vi "MecaOdometry_Update.vi"(8 "WheelSpeeds":T8 {"RearRightSpeed" format="%19.3f"; "RearLeftSpeed" format="%19.3f"; "FrontRightSpeed" format="%19.3f"; "FrontLeftSpeed" format="%19.3f"}, 9 "GyroAngle":T4={"VALUE"=0.0, "COS"=1.0, "SIN"=0.0} {"SIN" format="%13.4f"; "COS" format="%13.4f"; "VALUE" format="%13.4f"}, 10 "Time":dbl=-1.0 format="%33.4f", 11 "in MECA_DRIVE_ODOMETRY":T1={"POSE"={"TRANSLATION"={"X"=0.0, "Y"=0.0}, "ROTATION"={"VALUE"=0.0, "COS"=1.0, "SIN"=0.0}}, "PrevTime"=0.0, "GyroOffset"={"VALUE"=0.0, "COS"=0.0, "SIN"=0.0}, "PreviousAngle"={"VALUE"=0.0, "COS"=0.0, "SIN"=0.0}, "Kinematics"={"FrontLeft"={"X"=0.0, "Y"=0.0}, "FrontRight"={"X"=0.0, "Y"=0.0}, "RearLeft"={"X"=0.0, "Y"=0.0}, "RearRight"={"X"=0.0, "Y"=0.0}, "InverseKinematics"=[[0.0, 1.0, -1.0, 0.0], [0.0, 1.0, 1.0, 0.0], [0.0, 1.0, 1.0, 0.0], [0.0, 1.0, -1.0, 0.0]], "ForwardKinematics"=[[0.0, 1.0, -1.0, 0.0], [0.0, 1.0, 1.0, 0.0], [0.0, 1.0, 1.0, 0.0], [0.0, 1.0, -1.0, 0.0]], "PrevCoR"={"X"=0.0, "Y"=0.0}}, "PreviousWheelPositions"={"FrontLeft"=0.0, "FrontRight"=0.0, "RearLeft"=0.0, "RearRight"=0.0}} {"PreviousWheelPositions"."RearRight" format="%19.3f"; "PreviousWheelPositions"."RearLeft" format="%19.3f"; "PreviousWheelPositions"."FrontRight" format="%19.3f"; "PreviousWheelPositions"."FrontLeft" format="%19.3f"; "Kinematics"."PrevCoR"."Y" format="%14.3f"; "Kinematics"."PrevCoR"."X" format="%14.3f"; "Kinematics"."RearRight"."Y" format="%14.3f"; "Kinematics"."RearRight"."X" format="%14.3f"; "Kinematics"."RearLeft"."Y" format="%14.3f"; "Kinematics"."RearLeft"."X" format="%14.3f"; "Kinematics"."FrontRight"."Y" format="%14.3f"; "Kinematics"."FrontRight"."X" format="%14.3f"; "Kinematics"."FrontLeft"."Y" format="%14.3f"; "Kinematics"."FrontLeft"."X" format="%14.3f"; "PreviousAngle"."SIN" format="%13.4f"; "PreviousAngle"."COS" format="%13.4f"; "PreviousAngle"."VALUE" format="%13.4f"; "GyroOffset"."SIN" format="%13.4f"; "GyroOffset"."COS" format="%13.4f"; "GyroOffset"."VALUE" format="%13.4f"; "PrevTime" format="%13.4f"; "POSE"."ROTATION"."SIN" format="%13.4f"; "POSE"."ROTATION"."COS" format="%13.4f"; "POSE"."ROTATION"."VALUE" format="%13.4f"; "POSE"."TRANSLATION"."Y" format="%14.3f"; "POSE"."TRANSLATION"."X" format="%14.3f"}) -> (1 "POSE":T2={"TRANSLATION"={"X"=0.0, "Y"=0.0}, "ROTATION"={"VALUE"=0.0, "COS"=1.0, "SIN"=0.0}} {"ROTATION"."SIN" format="%13.4f"; "ROTATION"."COS" format="%13.4f"; "ROTATION"."VALUE" format="%13.4f"; "TRANSLATION"."Y" format="%14.3f"; "TRANSLATION"."X" format="%14.3f"}, 3 "out MECA_DRIVE_ODOMETRY":T1={"POSE"={"TRANSLATION"={"X"=0.0, "Y"=0.0}, "ROTATION"={"VALUE"=0.0, "COS"=1.0, "SIN"=0.0}}, "PrevTime"=0.0, "GyroOffset"={"VALUE"=0.0, "COS"=0.0, "SIN"=0.0}, "PreviousAngle"={"VALUE"=0.0, "COS"=0.0, "SIN"=0.0}, "Kinematics"={"FrontLeft"={"X"=0.0, "Y"=0.0}, "FrontRight"={"X"=0.0, "Y"=0.0}, "RearLeft"={"X"=0.0, "Y"=0.0}, "RearRight"={"X"=0.0, "Y"=0.0}, "InverseKinematics"=[[0.0, 1.0, -1.0, 0.0], [0.0, 1.0, 1.0, 0.0], [0.0, 1.0, 1.0, 0.0], [0.0, 1.0, -1.0, 0.0]], "ForwardKinematics"=[[0.0, 1.0, -1.0, 0.0], [0.0, 1.0, 1.0, 0.0], [0.0, 1.0, 1.0, 0.0], [0.0, 1.0, -1.0, 0.0]], "PrevCoR"={"X"=0.0, "Y"=0.0}}, "PreviousWheelPositions"={"FrontLeft"=0.0, "FrontRight"=0.0, "RearLeft"=0.0, "RearRight"=0.0}} {"PreviousWheelPositions"."RearRight" format="%19.3f"; "PreviousWheelPositions"."RearLeft" format="%19.3f"; "PreviousWheelPositions"."FrontRight" format="%19.3f"; "PreviousWheelPositions"."FrontLeft" format="%19.3f"; "Kinematics"."PrevCoR"."Y" format="%14.3f"; "Kinematics"."PrevCoR"."X" format="%14.3f"; "Kinematics"."RearRight"."Y" format="%14.3f"; "Kinematics"."RearRight"."X" format="%14.3f"; "Kinematics"."RearLeft"."Y" format="%14.3f"; "Kinematics"."RearLeft"."X" format="%14.3f"; "Kinematics"."FrontRight"."Y" format="%14.3f"; "Kinematics"."FrontRight"."X" format="%14.3f"; "Kinematics"."FrontLeft"."Y" format="%14.3f"; "Kinematics"."FrontLeft"."X" format="%14.3f"; "PreviousAngle"."SIN" format="%13.4f"; "PreviousAngle"."COS" format="%13.4f"; "PreviousAngle"."VALUE" format="%13.4f"; "GyroOffset"."SIN" format="%13.4f"; "GyroOffset"."COS" format="%13.4f"; "GyroOffset"."VALUE" format="%13.4f"; "PrevTime" format="%13.4f"; "POSE"."ROTATION"."SIN" format="%13.4f"; "POSE"."ROTATION"."COS" format="%13.4f"; "POSE"."ROTATION"."VALUE" format="%13.4f"; "POSE"."TRANSLATION"."Y" format="%14.3f"; "POSE"."TRANSLATION"."X" format="%14.3f"})   [LabVIEW 2019]
doc: "Updates the robot's position on the field using forward kinematics and integration of the pose over time. This method automatically calculates the current time to calculate period (difference between two timestamps). The period is used to calculate the change in distance from a velocity. This also takes in an angle parameter which is used instead of the angular rate that is calculated from forward kinematics.\n\nThis method uses the FPGA time.\n \nParameters:\n - MecaDriveOdometry - Data structure\n - Time -- Current time in seconds (Optional)\n - gyroAngle - The angle reported by the gyroscope.\n - wheelSpeeds - The current wheel speeds.\n\nReturns:\n - MecaDriveOdometry - Updated data structure\n - Pose - The new pose of the robot."
uses:
  TypeDef/MECA_DRIVE_ODOMETRY.ctl
  TypeDef/POSE2D.ctl
  TypeDef/TRANSLATION2D.ctl
  TypeDef/ROTATION2D.ctl
  TypeDef/MECA_DRIVE_KINEMATICS.ctl
  <vilib>/Analysis/Matrix/Datatypes/RealMatrix.ctl
  TypeDef/MECA_WHEEL_POSITIONS.ctl
  TypeDef/MECA_WHEEL_SPEEDS.ctl
  Trajectory_Library.lvlib
  <vilib>/Analysis/Matrix/NI_Matrix.lvlib
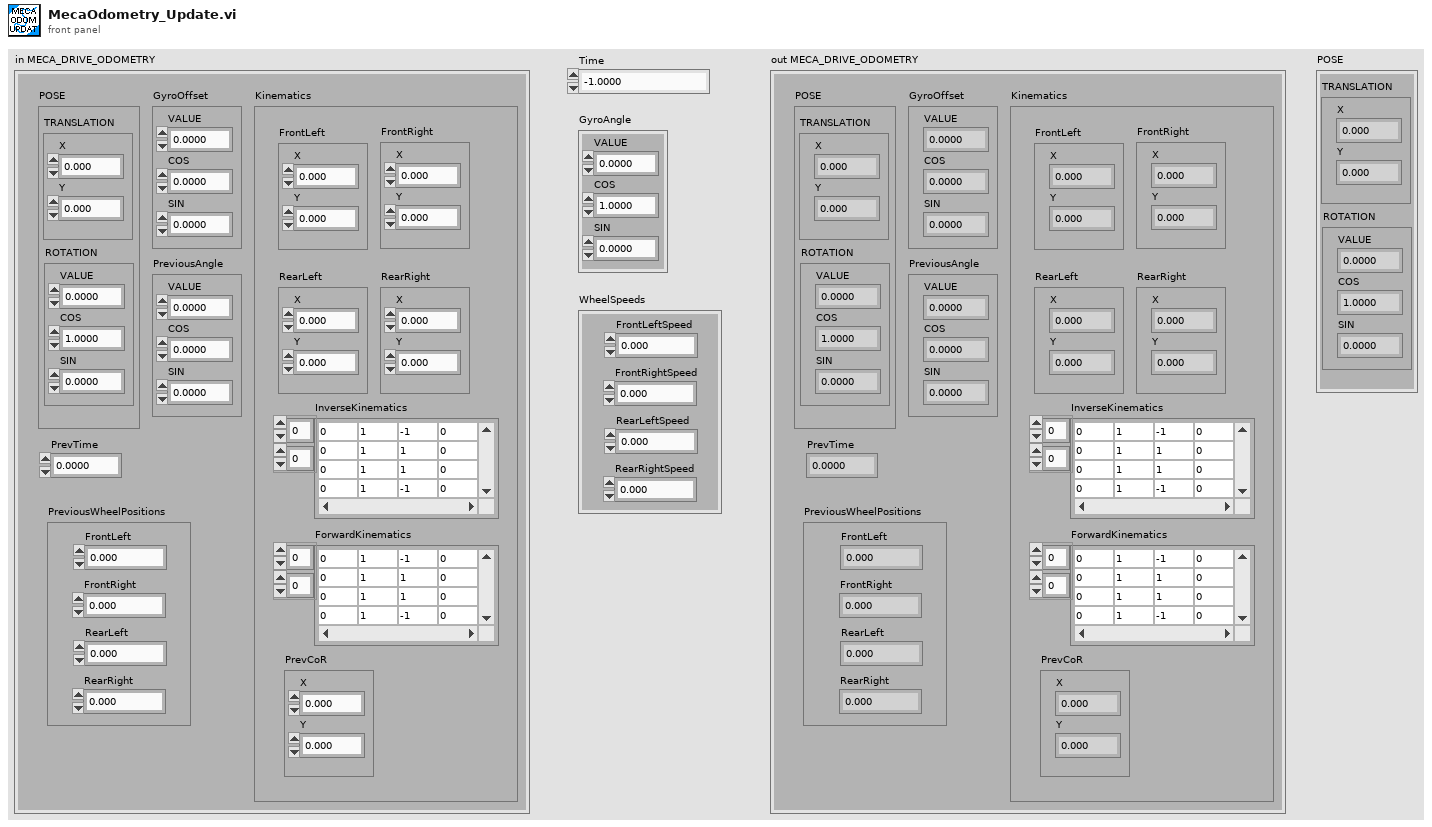
[diagram p1: front panel]
types:
  T1 = typedef "Trajectory_Library.lvlib/MECA_DRIVE_ODOMETRY.ctl" = cluster{"POSE":T2, "PrevTime":dbl, "GyroOffset":T4, "PreviousAngle":T4, "Kinematics":T5, "PreviousWheelPositions":T7}
  T2 = typedef "Trajectory_Library.lvlib/POSE2D.ctl" = cluster{"TRANSLATION":T3, "ROTATION":T4}
  T3 = typedef "Trajectory_Library.lvlib/TRANSLATION2D.ctl" = cluster{"X":dbl, "Y":dbl}
  T4 = typedef "Trajectory_Library.lvlib/ROTATION2D.ctl" = cluster{"VALUE":dbl, "COS":dbl, "SIN":dbl}
  T5 = typedef "Trajectory_Library.lvlib/MECA_DRIVE_KINEMATICS.ctl" = cluster{"FrontLeft":T3, "FrontRight":T3, "RearLeft":T3, "RearRight":T3, "InverseKinematics":T6, "ForwardKinematics":T6, "PrevCoR":T3}
  T6 = typedef "NI_Matrix.lvlib/RealMatrix.ctl" = dbl[][]
  T7 = typedef "Trajectory_Library.lvlib/MECA_WHEEL_POSITIONS.ctl" = cluster{"FrontLeft":dbl, "FrontRight":dbl, "RearLeft":dbl, "RearRight":dbl}
  T8 = typedef "Trajectory_Library.lvlib/MECA_WHEEL_SPEEDS.ctl" = cluster{"FrontLeftSpeed":dbl, "FrontRightSpeed":dbl, "RearLeftSpeed":dbl, "RearRightSpeed":dbl}
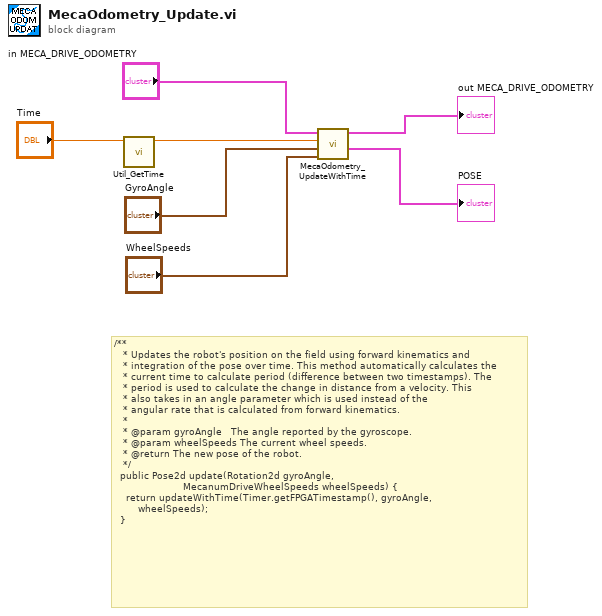
[diagram p0: block diagram]
diagram:
  # "/**\n   * Updates the robot's position on the field using forward kinematics and\n   * integration of the pose over time. This method automatically calculates the\n   * current time to calculate period (difference between two timestamps). The\n   * period is used to calculate the change in distance from a velocity. This\n   * also takes in an angle parameter which is used instead of the\n   * angular rate that is calculated from forward kinematics.\n   *\n   * @param gyroAngle   The angle reported by the gyroscope.\n   * @param wheelSpeeds The current wheel speeds.\n   * @return The new pose of the robot.\n   */\n  public Pose2d update(Rotation2d gyroAngle,\n                       MecanumDriveWheelSpeeds wheelSpeeds) {\n    return updateWithTime(Timer.getFPGATimestamp(), gyroAngle,\n        wheelSpeeds);\n  }"
  n1 = call "Util_GetTime.vi"("Pass_Through_Time"="Time") -> ("FPGA_Time_Seconds"=w6:dbl)  [unwired: 9 in, 1 out]
  n2 = call "MecaOdometry_UpdateWithTime.vi"("WheelSpeeds"="WheelSpeeds", "GyroAngle"="GyroAngle", "CurrentTime"=w6, "in MECA_DRIVE_ODOMETRY"="in MECA_DRIVE_ODOMETRY") -> ("POSE"=→"POSE":T2, "out MECA_DRIVE_ODOMETRY"=→"out MECA_DRIVE_ODOMETRY":T1)  [unwired: 6 in]
